vi "record selected tracks.vi"(6 "index":i32, 7 "Track Controls":T2 {"Track 3"."Volume Settings"."Volume" scale=0.001..5.0; "Track 3"."Volume Settings"."Pan" scale=0.0..1.0; "Track 3"."Effects Settings"."Delay 2" scale=0.0..10.0; "Track 3"."Effects Settings"."Delay" scale=0.0..10.0; "Track 2"."Volume Settings"."Volume" scale=0.001..5.0; "Track 2"."Volume Settings"."Pan" scale=0.0..1.0; "Track 2"."Effects Settings"."Delay 2" scale=0.0..10.0; "Track 2"."Effects Settings"."Delay" scale=0.0..10.0; "Track 1"."Volume Settings"."Volume" scale=0.001..5.0; "Track 1"."Volume Settings"."Pan" scale=0.0..1.0; "Track 1"."Effects Settings"."Delay 2" scale=0.0..10.0; "Track 1"."Effects Settings"."Delay" scale=0.0..10.0; "Track 0"."Volume Settings"."Volume" scale=0.001..5.0; "Track 0"."Volume Settings"."Pan" scale=0.0..1.0; "Track 0"."Effects Settings"."Delay 2" scale=0.0..10.0; "Track 0"."Effects Settings"."Delay" scale=0.0..10.0}, 8 "Blank Track":T1, 9 "AudioIn/Right (N Samples)":dbl[](array[numeric]), 10 "AudioIn/Left (N Samples)":dbl[](array[numeric]), 11 "4-Track Audio in":T6) -> (3 "4-Track Audio out":T6)   [LabVIEW 2014]
uses:
  Controls/4 Track Audio.ctl
  Controls/Audio In.ctl
  Controls/Track Controls.ctl
  Controls/Track Settings.ctl
  Controls/Track Effects Settings.ctl
  Controls/Track Volume Settings.ctl
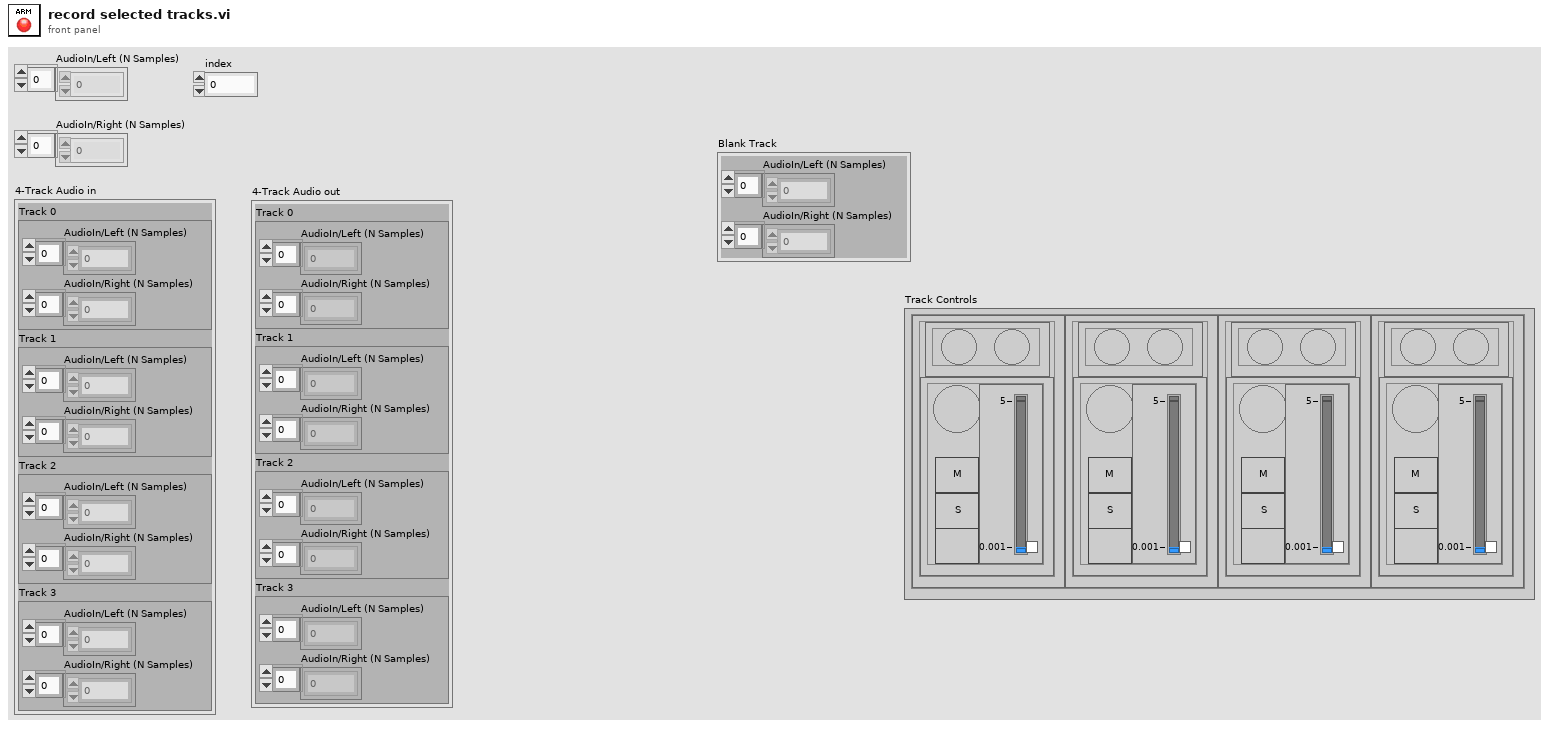
[diagram p1: front panel]
types:
  T1 = typedef "Audio In.ctl" = cluster{"AudioIn/Left (N Samples)":dbl[], "AudioIn/Right (N Samples)":dbl[]}
  T2 = typedef "Track Controls.ctl" = cluster{"Track 0":T3, "Track 1":T3, "Track 2":T3, "Track 3":T3}
  T3 = typedef "Track Settings.ctl" = cluster{"Effects Settings":T4, "Volume Settings":T5}
  T4 = typedef "Track Effects Settings.ctl" = cluster{"Delay":dbl, "Delay 2":dbl}
  T5 = typedef "Track Volume Settings.ctl" = cluster{"Mute":bool, "Solo":bool, "Record":bool, "Pan":dbl, "Volume":dbl}
  T6 = typedef "4 Track Audio.ctl" = cluster{"Track 0":T1, "Track 1":T1, "Track 2":T1, "Track 3":T1}
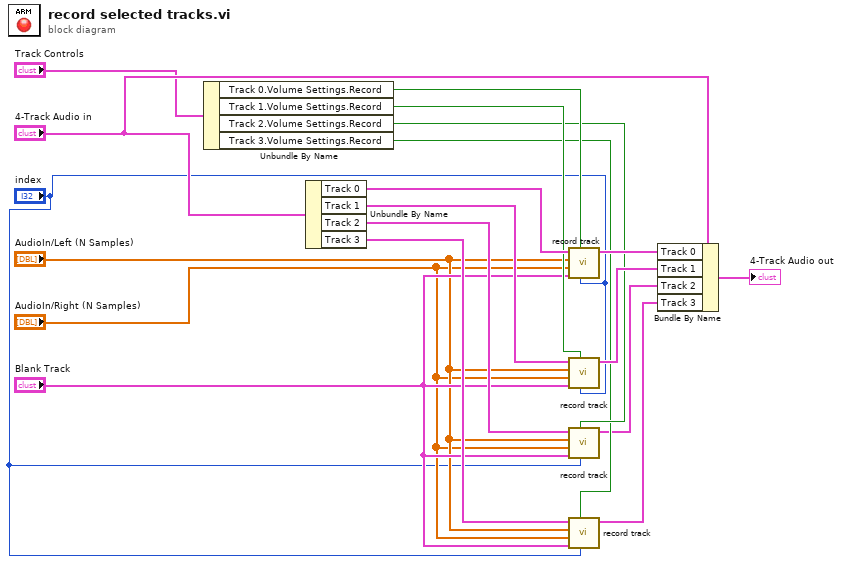
[diagram p0: block diagram]
diagram:
  n1 = Unbundle By Name("Track Controls") -> ("Track 0.Volume Settings.Record"=w15:bool, "Track 1.Volume Settings.Record"=w13:bool, "Track 2.Volume Settings.Record"=w10:bool, "Track 3.Volume Settings.Record"=w8:bool)
  n2 = Unbundle By Name("4-Track Audio in") -> ("Track 0"=w14:T1, "Track 1"=w12:T1, "Track 2"=w9:T1, "Track 3"=w7:T1)
  n3 = call "record track.vi"("index"="index", "Record"=w15, "Blank Track"="Blank Track", "AudioIn/Right (N Samples)"="AudioIn/Right (N Samples)", "AudioIn/Left (N Samples)"="AudioIn/Left (N Samples)", "Track In"=w14) -> ("Track Out"=w16:T1)  [unwired: 5 in]
  n4 = call "record track.vi"("index"="index", "Record"=w13, "Blank Track"="Blank Track", "AudioIn/Right (N Samples)"="AudioIn/Right (N Samples)", "AudioIn/Left (N Samples)"="AudioIn/Left (N Samples)", "Track In"=w12) -> ("Track Out"=w11:T1)  [unwired: 5 in]
  n5 = call "record track.vi"("index"="index", "Record"=w10, "Blank Track"="Blank Track", "AudioIn/Right (N Samples)"="AudioIn/Right (N Samples)", "AudioIn/Left (N Samples)"="AudioIn/Left (N Samples)", "Track In"=w9) -> ("Track Out"=w6:T1)  [unwired: 5 in]
  n6 = call "record track.vi"("index"="index", "Record"=w8, "Blank Track"="Blank Track", "AudioIn/Right (N Samples)"="AudioIn/Right (N Samples)", "AudioIn/Left (N Samples)"="AudioIn/Left (N Samples)", "Track In"=w7) -> ("Track Out"=w5:T1)  [unwired: 5 in]
  n7 = Bundle By Name(cluster="4-Track Audio in", "Track 0"=w16, "Track 1"=w11, "Track 2"=w6, "Track 3"=w5) -> (→"4-Track Audio out":T6)
